vi "example_error_bypass.vi"   [LabVIEW 2015]
uses:
  polys/poly_error_bypass_out.vi
  polys/poly_error_bypass_in.vi
  merge_errors.vi
  polys/poly_merge_errors_up.vi
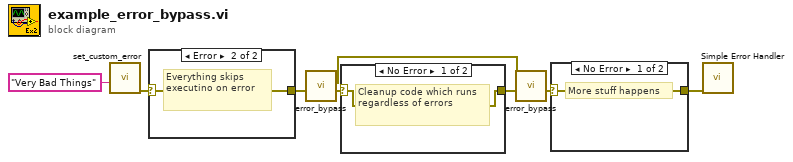
[diagram p0: block diagram]
diagram:
  n1 = call "set_custom_error.vi"("custom error description"="Very Bad Things" ("source")) -> ("error out"=w1:errorcluster)  [unwired: 10 in]
  n2 = case shown="Error" w1 {
    selector: w1 -> [w9 w10]
    tunnel: [w9 w10] -> w5
    frame No Error {
      # "Normal working case"
    }
    frame Error {
      # "Everything skips executino on error"
    }
  }
  n3 = call-poly "error_bypass.vi"("Error in"=w5) -> ("No error"=w7:errorcluster, "Error out"=w8:errorcluster)  [unwired: 9 in]
  n4 = case shown="No Error" w7 {
    selector: w7 -> [w11 w12]
    tunnel: [w11 w12] -> w6
    frame No Error {
      # "Cleanup code which runs regardless of errors"
    }
    frame Error {
    }
  }
  n5 = call-poly "error_bypass.vi"("Error in 2"=w6, "Error in"=w8) -> ("error out"=w4:errorcluster)  [unwired: 9 in]
  n6 = case shown="No Error" w4 {
    selector: w4 -> [w13 w14]
    tunnel: [w13 w14] -> w3
    frame No Error {
      # "More stuff happens"
    }
    frame Error {
      # "Or doesn't..."
    }
  }
  n7 = call <vilib>:"Simple Error Handler.vi"("error in (no error)"=w3) -> ()  [unwired: 4 in, 5 out]
